vi "Do Something.vi"(8 "error in (no error)":errorcluster, 10 "Bytes to Read":i32, 11 "Inst.TSL210 in":refnum<class "Inst.TSL210.lvclass">) -> (0 "error out":errorcluster, 3 "Inst.TSL210 out":refnum<class "Inst.TSL210.lvclass">)   [LabVIEW 2019, in "Inst.TSL210.lvclass"]
uses:
  Inst.TSL210.lvclass
  C:/Program Files (x86)/National Instruments/LabVIEW 2019/user.lib/LevyLab/Instrument Framework/SMOs/Instrument/Instrument.lvclass
  Typedefs/Inst.TSL210.Commands--Enum.ctl
  <userlib>/LevyLab/Instrument Framework/SMOs/Instrument/Instrument.lvclass/Instrument.ctl
  67792bfe-8e2c-4879-abc2-cb448bcec168.vi
  67792bfe-8e2c-4879-abc2-cb448bcec168.vi/e6734212-7c9e-4ce8-a442-683b18d6b7e6.vi
  <userlib>/LevyLab/Instrument Framework/SMOs/Instrument/API/Send and Receive.vi
  67792bfe-8e2c-4879-abc2-cb448bcec168.vi/d08038f8-4acd-46a3-976f-e1cbe8915b66.vi
  <userlib>/LevyLab/Instrument Framework/SMOs/Instrument/Private/Get Client Type.vi
  67792bfe-8e2c-4879-abc2-cb448bcec168.vi/e6734212-7c9e-4ce8-a442-683b18d6b7e6.vi/c45d00ac-9d04-46c9-a4f5-b0dcc005fc38.vi
  67792bfe-8e2c-4879-abc2-cb448bcec168.vi/e6734212-7c9e-4ce8-a442-683b18d6b7e6.vi/98b85601-7043-4932-8313-ea7ea4f11616.vi
  67792bfe-8e2c-4879-abc2-cb448bcec168.vi/d08038f8-4acd-46a3-976f-e1cbe8915b66.vi/800cf9c4-7383-40cf-9bc6-eb11c7b09f2f.vi
  67792bfe-8e2c-4879-abc2-cb448bcec168.vi/d08038f8-4acd-46a3-976f-e1cbe8915b66.vi/0f5049b1-9107-4d80-b470-81422f3edf74.vi
  67792bfe-8e2c-4879-abc2-cb448bcec168.vi/d08038f8-4acd-46a3-976f-e1cbe8915b66.vi/800cf9c4-7383-40cf-9bc6-eb11c7b09f2f.vi/fadd8450-4042-4d20-8257-693326a0ff50.vi
  67792bfe-8e2c-4879-abc2-cb448bcec168.vi/d08038f8-4acd-46a3-976f-e1cbe8915b66.vi/800cf9c4-7383-40cf-9bc6-eb11c7b09f2f.vi/1fd9aa42-e19b-4fc1-b3df-051849edd69a.vi
  <userlib>/LevyLab/Instrument Framework/SMOs/Instrument/Private/Get RC Connection Status.vi
  <userlib>/LevyLab/Instrument Framework/SMOs/Instrument/API/Enum to String.vi
  <userlib>/LevyLab/Instrument Framework/SMOs/RemoteControl/API/Send and Receive.vi
  <vilib>/Utility/Data Type/Get Type Information.vi
  <vilib>/JDP Science/JSONtext/JSON text to Variant.vi
  <userlib>/LevyLab/Instrument Framework/SMOs/Instrument/API/Instrument.GetPublicEvents.vi
  <vilib>/JDP Science/JSONtext/Variant to JSON Text.vi
  <vilib>/National Instruments/GUID Generator/Guid Generator.vi
  <userlib>/LevyLab/Instrument Framework/SMOs/Instrument/API/Instrument.MessageToProcess.vi
  <userlib>/LevyLab/Instrument Framework/SMOs/Instrument/Private/Instrument.MessageFromProcess.EventStructure.vi
  <vilib>/JDP Science/JSONtext/LVClass Serializer/JSONtext LVClass Serializer.lvclass
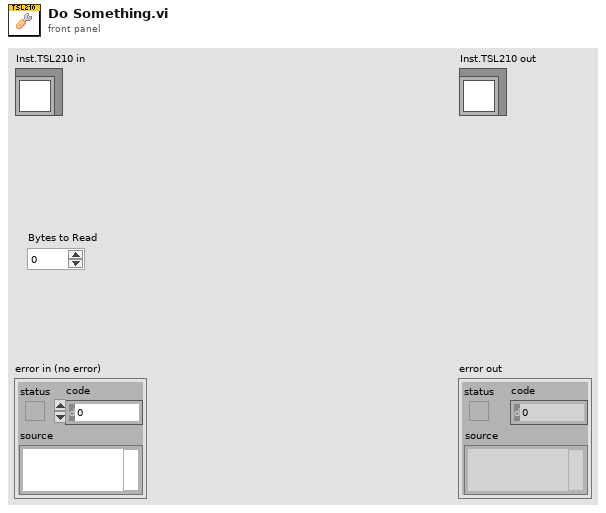
[diagram p1: front panel]
types:
  T1 = typedef "Inst.TSL210.lvclass/Inst.TSL210.Commands--Enum.ctl" = enum16{"Do Something"}
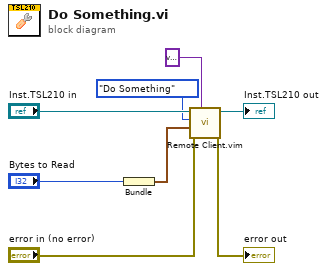
[diagram p0: block diagram]
diagram:
  n1 = Bundle("Bytes to Read"="Bytes to Read") -> (w2:cluster{"Bytes to Read":i32})  [unwired: 1 in]
  n2 = call "Remote Client.vim"("Data Out type"=variant, "error in (no error)"="error in (no error)", "params"=w2, "method"=Inst.TSL210.Commands--Enum."Do Something" ("Commands"), "Instrument in"="Inst.TSL210 in") -> ("error out"=→"error out":errorcluster, "Instrument out"=→"Inst.TSL210 out":refnum<class "Inst.TSL210.lvclass">)  [unwired: 3 in, 2 out]
